vi "regextest.vi"(11 "Molecule":string) -> (1 "Elements":string[](array[string]), 2 "array":string[][](array[string]), 3 "Numbers":i32[](array[numeric]))   [LabVIEW 2023]
uses:
  <vilib>/regexp/Match Regular Expression.xnode
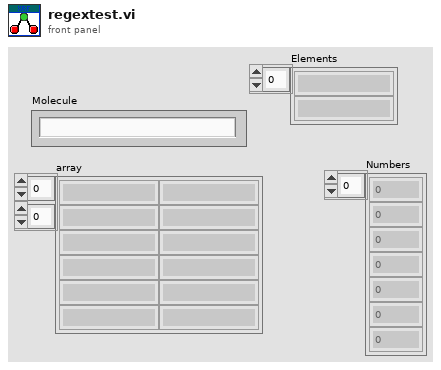
[diagram p1: front panel]
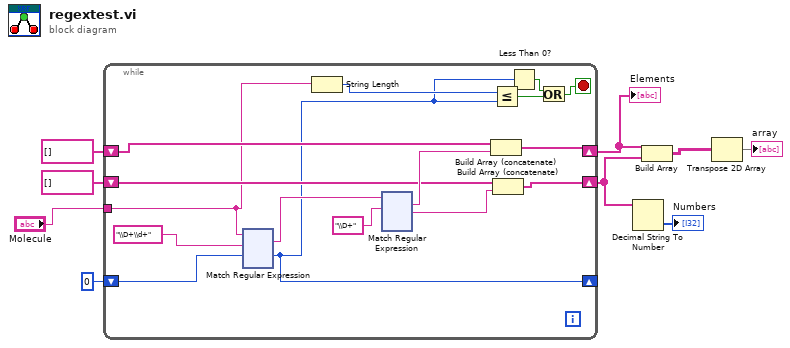
[diagram p0: block diagram]
diagram:
  n1 = while {
    shift-right: [w14] -> _
    shift-left: 0 ("offset past match") -> [w24]
    shift-right: [w10] -> w9
    shift-left: string[] [] -> [w20]
    shift-right: [w16] -> w2
    shift-left: string[] [] -> [w18]
    tunnel: "Molecule" -> [w15]
    stop <- w11 stop-if-true
    n2 = xnode "Match Regular Expression"("input string"=w15, "regular expression"="\\D+\\d+" ("regex"), "offset (0)"=w24) -> ("whole match"=w21:string, "offset past match"=w14:i32)  [unwired: 3 in, 3 out]
    n3 = String Length(string=w15) -> (length=w23:i32)
    n4 = xnode "Match Regular Expression"("input string"=w21, "regular expression"="\\D+") -> ("whole match"=w19:string, "after match"=w17:string)  [unwired: 4 in, 3 out]
    n5 = Build Array (concatenate)(w20, w19) -> (w10:string[])
    n6 = Less Or Equal?(x=w23, y=w14) -> (x <= y?=w12:bool)
    n7 = Build Array (concatenate)(w18, w17) -> (w16:string[])
    n8 = Less Than 0?(x=w14) -> (x < 0?=w13:bool)
    n9 = Or(x=w13, y=w12) -> (x .or. y?=w11:bool)
  }
  "Elements" <- w9
  n10 = Decimal String To Number(string=w2) -> (number=→"Numbers":i32[])  [unwired: 2 in, 1 out]
  n11 = Build Array(w9, w2) -> (w8:string[][])
  n12 = Transpose 2D Array(2D array=w8) -> (transposed array=→"array":string[][])
